vi "TematyDane_new.vi"(9 "Value":u16, 10 "TematyDane in":string[][](array[string])) -> (0 "Array":i32[](array[numeric]), 1 "Dane":string[](array[string]), 2 "Podtemat":string, 3 "Temat":string)   [LabVIEW 2017]
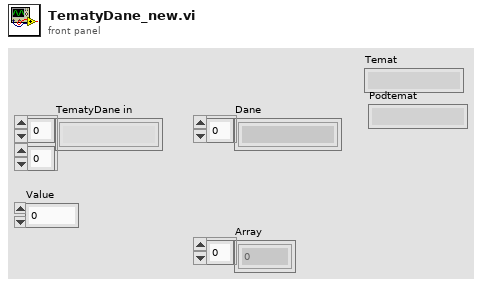
[diagram p1: front panel]
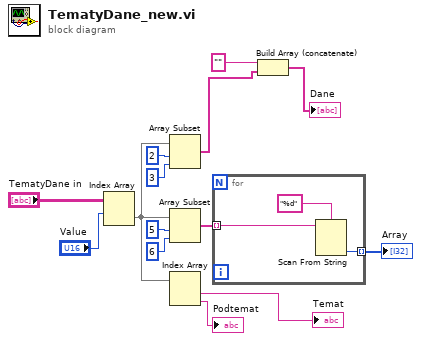
[diagram p0: block diagram]
diagram:
  n1 = Index Array(array="TematyDane in", index (row)="Value") -> (element=w6:string[])  [unwired: 1 in]
  n2 = Array Subset(array=w6, index=2, length=3) -> (w2:string[])
  n3 = Array Subset(array=w6, index=5, length=6) -> (w11:string[])
  n4 = Index Array(array=w6) -> (element #1=→"Temat":string, element #2=→"Podtemat":string)  [unwired: 2 in]
  n5 = for {
    tunnel: w11 -> [w17] mode=indexing
    tunnel: [w16] -> w12 mode=indexing
    n6 = Scan From String(format string="%d", input string=w17) -> (output 1=w16:i32)  [unwired: 3 in, 3 out]
  }
  "Array" <- w12
  n7 = Build Array (concatenate)("" ("format string"), w2) -> (→"Dane":string[])
